vi "Set Camera Configuration.vi"(8 "error in (no error)":errorcluster, 11 "CCDCamera in":refnum<class "Ixon_Ultra.lvclass">) -> (0 "error out":errorcluster, 3 "CCDCamera out":refnum<class "Ixon_Ultra.lvclass">)   [LabVIEW 2018, in "Ixon_Ultra.lvclass"]
doc: "Set the camera configuration\n\nThis function records the given operating parameters in the camera. However, the parameters will only bewritten if their last value is different from the most recent one."
uses:
  Ixon_Ultra.lvclass
  C:/Users/Denis/Desktop/S4ACS/S4ACS/Simulated_CCD_Camera/Simulated Camera.lvclass
  Simulated_CCD_Camera/Simulated Camera.lvclass
panel:
  out "x != y?":T1
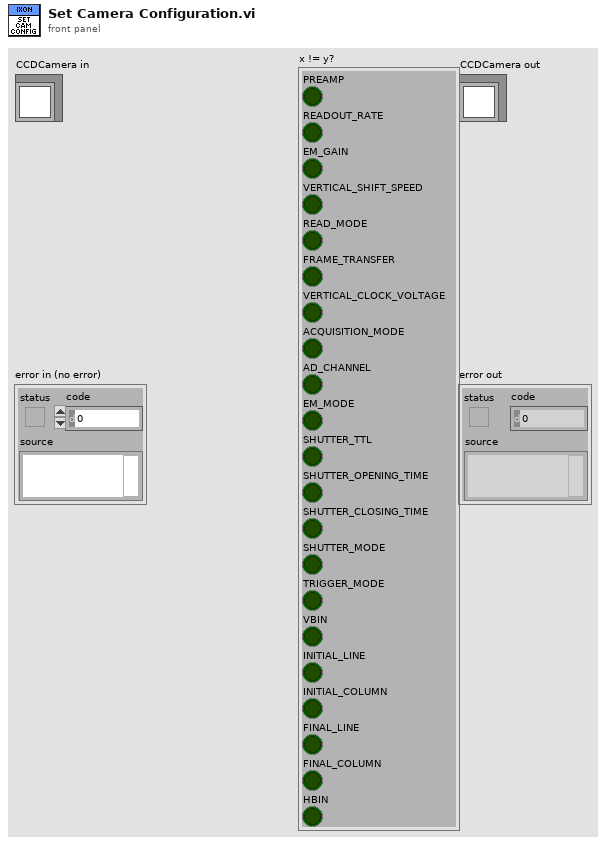
[diagram p1: front panel]
types:
  T1 = cluster{"PREAMP":bool, "READOUT_RATE":bool, "EM_GAIN":bool, "VERTICAL_SHIFT_SPEED":bool, "READ_MODE":bool, "FRAME_TRANSFER":bool, "VERTICAL_CLOCK_VOLTAGE":bool, "ACQUISITION_MODE":bool, "AD_CHANNEL":bool, "EM_MODE":bool, "SHUTTER_TTL":bool, "SHUTTER_OPENING_TIME":bool, "SHUTTER_CLOSING_TIME":bool, "SHUTTER_MODE":bool, "TRIGGER_MODE":bool, "VBIN":bool, "INITIAL_LINE":bool, "INITIAL_COLUMN":bool, "FINAL_LINE":bool, "FINAL_COLUMN":bool, "HBIN":bool}
  T2 = cluster{"PREAMP":u16, "READOUT_RATE":u16, "EM_GAIN":u16, "VERTICAL_SHIFT_SPEED":u16, "READ_MODE":u16, "FRAME_TRANSFER":bool, "VERTICAL_CLOCK_VOLTAGE":u16, "ACQUISITION_MODE":u16, "AD_CHANNEL":u16, "EM_MODE":u16, "SHUTTER_TTL":u16, "SHUTTER_OPENING_TIME":u16, "SHUTTER_CLOSING_TIME":u16, "SHUTTER_MODE":u16, "TRIGGER_MODE":u16, "VBIN":u16, "INITIAL_LINE":u16, "INITIAL_COLUMN":u16, "FINAL_LINE":u16, "FINAL_COLUMN":u16, "HBIN":u16}
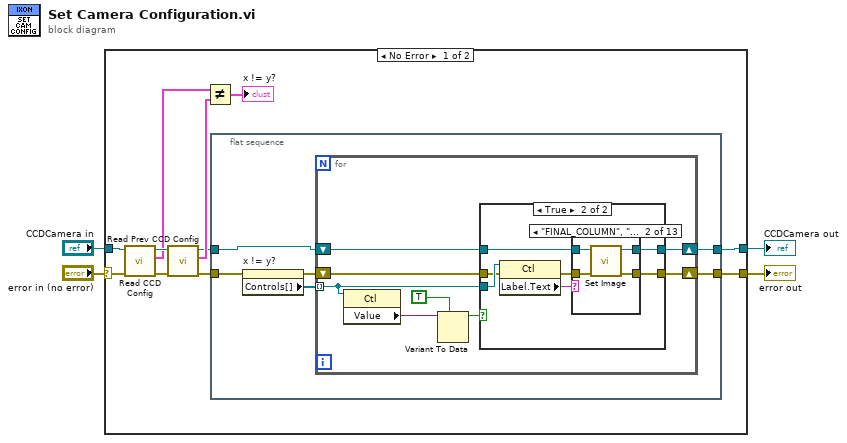
[diagram p0: block diagram]
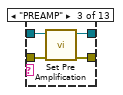
[diagram p4: hidden frame]
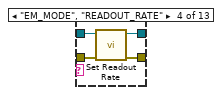
[diagram p5: hidden frame]
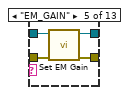
[diagram p6: hidden frame]
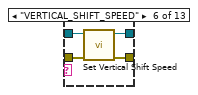
[diagram p7: hidden frame]
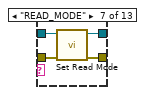
[diagram p8: hidden frame]
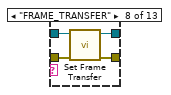
[diagram p9: hidden frame]
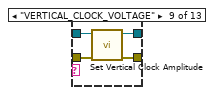
[diagram p10: hidden frame]
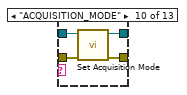
[diagram p11: hidden frame]
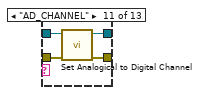
[diagram p12: hidden frame]
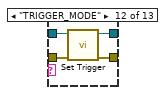
[diagram p13: hidden frame]
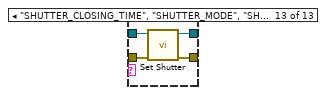
[diagram p14: hidden frame]
diagram:
  n1 = case shown="No Error" "error in (no error)" {
    selector: "error in (no error)" -> [w14 w90]
    tunnel: [w13 w90] -> w4
    tunnel: [w12 w89] -> w3
    tunnel: "CCDCamera in" -> [w11 w89]
    frame No Error {
      n2 = call "Read CCD Config.vi"("error in (no error)"=w14, "CCDCamera in"=w11) -> ("error out"=w8:errorcluster, "CCD Config"=w7:T2, "CCDCamera out"=w9:refnum<class "Ixon_Ultra.lvclass">)  [unwired: 7 in]
      n3 = call-dynamic "Read Prev CCD Config.vi"("error in (no error)"=w8, "Simulated_CCD_Camera in"=w9) -> ("error out"=w5:errorcluster, "Prev CCD Config"=w10:T2, "Simulated_CCD_Camera out"=w6:refnum<class "Ixon_Ultra.lvclass">)  [unwired: 7 in]
      n4 = Not Equal?(x=w7, y=w10) -> (x != y?=→"x != y?":T1)
      n5 = flat-sequence {
        tunnel: w5 -> [w16]
        tunnel: [w21] -> w13
        tunnel: w6 -> [w19]
        tunnel: [w18] -> w12
        frame #0 {
          n6 = property on="x != y?" class="Clust (strict)"(error in=w16) -> (error out=w20:errorcluster, "Controls[]"=w17:refnum<vi>[])  [unwired: 1 in, 1 out]
          n7 = for {
            tunnel: w17 -> [w28] mode=indexing
            shift-right: [w22] -> w21
            shift-left: w20 -> [w29]
            shift-right: [w23] -> w18
            shift-left: w19 -> [w24]
            n8 = property class="Ctl"(reference=w28) -> ("Value"=w27:variant)  [unwired: 1 in, 2 out]
            n9 = Variant To Data(type=TRUE, Variant=w27) -> (data=w25:bool)  [unwired: 1 in, 1 out]
            n10 = case shown="True" w25 {
              tunnel: w28 -> [_ w38]
              tunnel: [w31 w32] -> w22
              tunnel: w29 -> [w31 w36]
              tunnel: w24 -> [w30 w35]
              tunnel: [w30 w34] -> w23
              frame False {
              }
              frame True {
                n11 = property class="Ctl"(reference=w38, error in=w36) -> (error out=w33:errorcluster, "Label.Text"=w37:string)  [unwired: 1 out]
                n12 = case shown="\"FINAL_COLUMN\", \"FINAL_LINE\", \"HBIN\", \"INITIAL_COLUMN\", \"INITIAL_LINE\", \"VBIN\"" w37 {
                  tunnel: w35 -> [w40 w44 w48 w51 w56 w60 w64 w68 w71 w76 w80 w83 w88]
                  tunnel: [w40 w43 w47 w52 w55 w59 w63 w67 w72 w75 w79 w84 w87] -> w34
                  tunnel: w33 -> [w39 w42 w46 w50 w54 w58 w62 w66 w70 w74 w78 w82 w86]
                  tunnel: [w39 w41 w45 w49 w53 w57 w61 w65 w69 w73 w77 w81 w85] -> w32
                  frame "False", Default {
                  }
                  frame "FINAL_COLUMN", "FINAL_LINE", "HBIN", "INITIAL_COLUMN", "INITIAL_LINE", "VBIN" {
                    n13 = call-dynamic "Set Image.vi"("error in (no error)"=w42, "CCDCamera in"=w44) -> ("error out"=w41:errorcluster, "CCDCamera out"=w43:refnum<class "Ixon_Ultra.lvclass">)  [unwired: 8 in]
                  }
                  frame "PREAMP" {
                    n14 = call-dynamic "Set Pre Amplification.vi"("error in (no error)"=w46, "CCDCamera in"=w48) -> ("error out"=w45:errorcluster, "CCDCamera out"=w47:refnum<class "Ixon_Ultra.lvclass">)  [unwired: 8 in]
                  }
                  frame "EM_MODE", "READOUT_RATE" {
                    n15 = call-dynamic "Set Readout Rate.vi"("error in (no error)"=w50, "CCDCamera in"=w51) -> ("error out"=w49:errorcluster, "CCDCamera out"=w52:refnum<class "Ixon_Ultra.lvclass">)  [unwired: 8 in]
                  }
                  frame "EM_GAIN" {
                    n16 = call-dynamic "Set EM Gain.vi"("error in (no error)"=w54, "CCDCamera in"=w56) -> ("error out"=w53:errorcluster, "CCDCamera out"=w55:refnum<class "Ixon_Ultra.lvclass">)  [unwired: 8 in]
                  }
                  frame "VERTICAL_SHIFT_SPEED" {
                    n17 = call-dynamic "Set Vertical Shift Speed.vi"("error in (no error)"=w58, "CCDCamera in"=w60) -> ("error out"=w57:errorcluster, "CCDCamera out"=w59:refnum<class "Ixon_Ultra.lvclass">)  [unwired: 8 in]
                  }
                  frame "READ_MODE" {
                    n18 = call-dynamic "Set Read Mode.vi"("error in (no error)"=w62, "CCDCamera in"=w64) -> ("error out"=w61:errorcluster, "CCDCamera out"=w63:refnum<class "Ixon_Ultra.lvclass">)  [unwired: 8 in]
                  }
                  frame "FRAME_TRANSFER" {
                    n19 = call-dynamic "Set Frame Transfer.vi"("error in (no error)"=w66, "CCDCamera in"=w68) -> ("error out"=w65:errorcluster, "CCDCamera out"=w67:refnum<class "Ixon_Ultra.lvclass">)  [unwired: 8 in]
                  }
                  frame "VERTICAL_CLOCK_VOLTAGE" {
                    n20 = call-dynamic "Set Vertical Clock Amplitude.vi"("error in (no error)"=w70, "CCDCamera in"=w71) -> ("error out"=w69:errorcluster, "CCDCamera out"=w72:refnum<class "Ixon_Ultra.lvclass">)  [unwired: 8 in]
                  }
                  frame "ACQUISITION_MODE" {
                    n21 = call-dynamic "Set Acquisition Mode.vi"("error in (no error)"=w74, "CCDCamera in"=w76) -> ("error out"=w73:errorcluster, "CCDCamera out"=w75:refnum<class "Ixon_Ultra.lvclass">)  [unwired: 8 in]
                  }
                  frame "AD_CHANNEL" {
                    n22 = call-dynamic "Set Analogical to Digital Channel.vi"("error in (no error)"=w78, "CCDCamera in"=w80) -> ("error out"=w77:errorcluster, "CCDCamera out"=w79:refnum<class "Ixon_Ultra.lvclass">)  [unwired: 8 in]
                  }
                  frame "TRIGGER_MODE" {
                    n23 = call-dynamic "Set Trigger.vi"("error in (no error)"=w82, "CCDCamera in"=w83) -> ("error out"=w81:errorcluster, "CCDCamera out"=w84:refnum<class "Ixon_Ultra.lvclass">)  [unwired: 8 in]
                  }
                  frame "SHUTTER_CLOSING_TIME", "SHUTTER_MODE", "SHUTTER_OPENING_TIME", "SHUTTER_TTL" {
                    n24 = call-dynamic "Set Shutter.vi"("error in (no error)"=w86, "CCDCamera in"=w88) -> ("error out"=w85:errorcluster, "CCDCamera out"=w87:refnum<class "Ixon_Ultra.lvclass">)  [unwired: 8 in]
                  }
                }
              }
            }
          }
        }
      }
    }
    frame Error {
    }
  }
  "error out" <- w4
  "CCDCamera out" <- w3
